vi "Problem 4.vi"() -> (2 "Palindromes":i32[](array[numeric]), 3 "Largest Palindrome":i32)   [LabVIEW 2013, in "Problem 4.lvlib"]
uses:
  Problem 4.lvlib
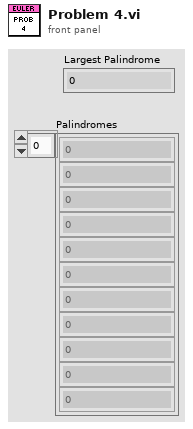
[diagram p1: front panel]
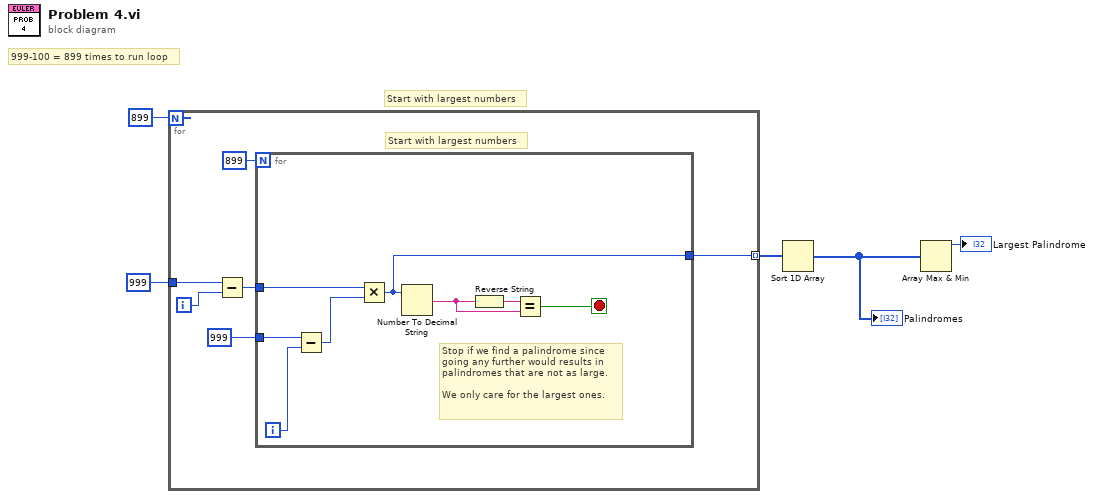
[diagram p0: block diagram]
diagram:
  # "Start with largest numbers"
  # "999-100 = 899 times to run loop"
  n1 = for {
    N: 899 -> [_]
    tunnel: 999 -> [w9]
    tunnel: [w6] -> w3 mode=indexing
    i -> [w8]
    # "Start with largest numbers"
    n2 = Subtract(x=w9, y=w8) -> (x-y=w7:i32)
    n3 = for {
      N: 899 -> [_]
      tunnel: 999 -> [w18]
      tunnel: w7 -> [w17]
      tunnel: [w12] -> w6
      i -> [w19]
      stop <- w13 stop-if-true
      # "Stop if we find a palindrome since\ngoing any further would results in\npalindromes that are not as large.\n\nWe only care for the largest ones."
      n4 = Subtract(x=w18, y=w19) -> (x-y=w16:i32)
      n5 = Multiply(x=w17, y=w16) -> (x*y=w12:i32)
      n6 = Number To Decimal String(number=w12) -> (decimal integer string=w14:string)  [unwired: 1 in]
      n7 = Reverse String(1:w14) -> (0:w15:string)
      n8 = Equal?(x=w15, y=w14) -> (x = y?=w13:bool)
    }
  }
  n9 = Sort 1D Array(array=w3) -> (sorted array=w2:i32[])
  "Palindromes" <- w2
  n10 = Array Max & Min(array=w2) -> (max value=→"Largest Palindrome":i32)  [unwired: 3 out]
